vi "Get Array Value at Index - Null.vi"(8 "error in (no error)":errorcluster, 10 "Index":i32, 11 "JSON Tree In (JSON Array)":variant) -> (0 "error out":errorcluster, 1 "is JSON Null?":bool, 2 "JSON Null Value":variant, 3 "JSON Tree Out Passthrough":variant)   [LabVIEW 2013, in "i3-json.lvlib"]
doc: "Use this template to build a VI to use as a subVI."
uses:
  i3-json.lvlib
  JSON Types/JSON Type.ctl
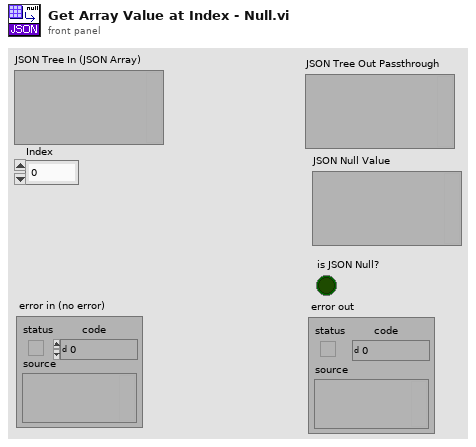
[diagram p1: front panel]
types:
  T1 = typedef "i3-json.lvlib/JSON Type.ctl" = enum8{"JSON Compatible", "JSON Array", "JSON Object", "JSON Null", "Double", "String", "Boolean", "Unknown", "Data JSON string"}
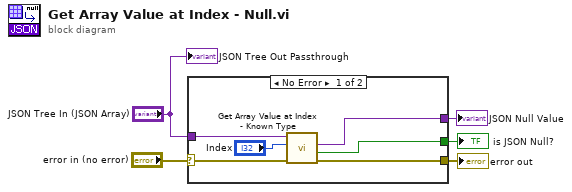
[diagram p0: block diagram]
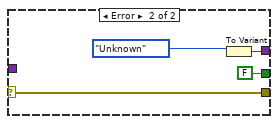
[diagram p2: hidden frame]
diagram:
  n1 = case shown="No Error" "error in (no error)" {
    selector: "error in (no error)" -> [w9 w15]
    tunnel: [w8 w15] -> w4
    tunnel: "JSON Tree In (JSON Array)" -> [w11 _]
    tunnel: [w7 FALSE ("is JSON Null?")] -> w3
    tunnel: [w6 w14] -> w2
    frame No Error {
      n2 = call "Get Array Value at Index - Known Type.vi"("error in (no error)"=w9, "Index"="Index", "JSON Tree In (JSON Array)"=w11) -> ("error out"=w8:errorcluster, "is JSON Null?"=w7:bool, "Value"=w6:variant)  [unwired: 3 in, 3 out]
    }
    frame Error {
      n3 = To Variant(anything=JSON_Type."Unknown" ("JSON Type")) -> (Variant=w14:variant)
    }
  }
  "error out" <- w4
  "is JSON Null?" <- w3
  "JSON Null Value" <- w2
  "JSON Tree Out Passthrough" <- "JSON Tree In (JSON Array)"
